vi "Joystick Values To Joystick Data.vi"(0 "Xbox Name":string="My Joystick RefNum", 3 "Left X3D Joystick Name":string="My Joystick RefNum", 5 "Right X3D Joystick Name":string="My Joystick RefNum") -> ()   [LabVIEW 2016]
uses:
  Joystick Global 6740.vi
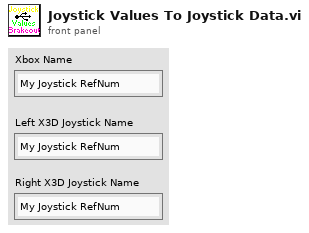
[diagram p1: front panel]
types:
  T1 = cluster{"A":bool, "B":bool, "X":bool, "Y":bool, "LB":bool, "RB":bool, "Back":bool, "Start":bool, "Left Joystick":bool, "Right Joystick":bool}
  T2 = cluster{"Left X":dbl, "Left Y":dbl, "Left Trigger":dbl, "Right Trigger":dbl, "Right X":dbl, "Right Y":dbl}
  T3 = cluster{"1":bool, "2":bool, "3":bool, "4":bool, "5":bool, "6":bool, "7":bool, "8":bool, "9":bool, "10":bool, "11":bool, "12":bool}
  T4 = cluster{"X Axis":dbl, "Y Axis":dbl, "Z Axis":dbl, "Slider":dbl}
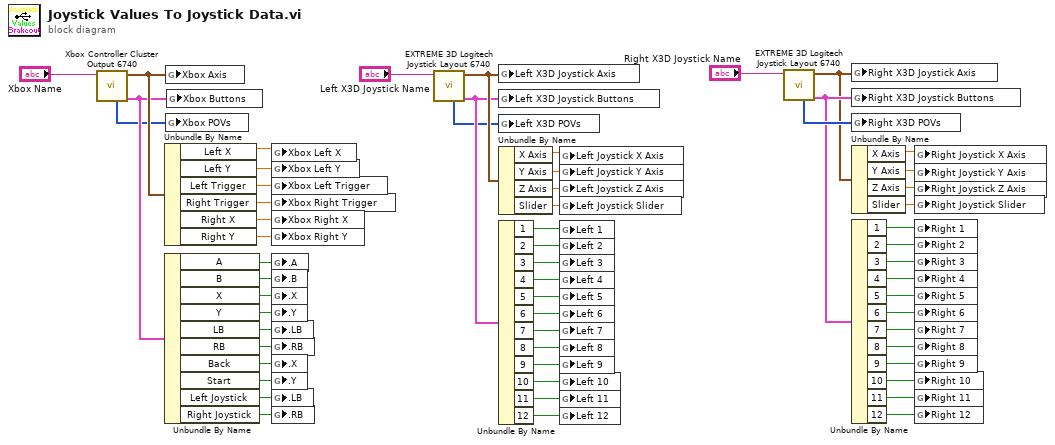
[diagram p0: block diagram]
diagram:
  n1 = call "Xbox Controller Cluster Output 6740.vi"("Joystick Name"="Xbox Name") -> ("Xbox Buttons"=w43:T1, "Xbox Axis"=w44:T2, "POVs"=w21:i16[])  [unwired: 8 in]
  n2 = Unbundle By Name(w44) -> ("Left X"=w60:dbl, "Left Y"=w59:dbl, "Left Trigger"=w58:dbl, "Right Trigger"=w57:dbl, "Right X"=w56:dbl, "Right Y"=w55:dbl)
  n3 = Unbundle By Name(w43) -> ("A"=w54:bool, "B"=w53:bool, "X"=w52:bool, "Y"=w51:bool, "LB"=w50:bool, "RB"=w49:bool, "Back"=w48:bool, "Start"=w47:bool, "Left Joystick"=w46:bool, "Right Joystick"=w45:bool)
  n4 = global write "Joystick Global 6740.vi" "Xbox Axis"(w44) -> ()
  n5 = global write "Joystick Global 6740.vi" "Xbox POVs"(w21) -> ()
  n6 = global write "Joystick Global 6740.vi" "Xbox Buttons"(w43) -> ()
  n7 = global write "Joystick Global 6740.vi" "Xbox Left X"(w60) -> ()
  n8 = global write "Joystick Global 6740.vi" "Xbox Left Y"(w59) -> ()
  n9 = global write "Joystick Global 6740.vi" "Xbox Left Trigger"(w58) -> ()
  n10 = global write "Joystick Global 6740.vi" "Xbox Right Trigger"(w57) -> ()
  n11 = global write "Joystick Global 6740.vi" "Xbox Right X"(w56) -> ()
  n12 = global write "Joystick Global 6740.vi" "Xbox Right Y"(w55) -> ()
  n13 = global write "Joystick Global 6740.vi" ".A"(w54) -> ()
  n14 = global write "Joystick Global 6740.vi" ".B"(w53) -> ()
  n15 = global write "Joystick Global 6740.vi" ".X"(w52) -> ()
  n16 = global write "Joystick Global 6740.vi" ".Y"(w51) -> ()
  n17 = global write "Joystick Global 6740.vi" ".LB"(w50) -> ()
  n18 = global write "Joystick Global 6740.vi" ".RB"(w49) -> ()
  n19 = global write "Joystick Global 6740.vi" ".X"(w48) -> ()
  n20 = global write "Joystick Global 6740.vi" ".Y"(w47) -> ()
  n21 = global write "Joystick Global 6740.vi" ".LB"(w46) -> ()
  n22 = global write "Joystick Global 6740.vi" ".RB"(w45) -> ()
  n23 = call "EXTREME 3D Logitech Joystick Layout 6740.vi"("Joystick Name"="Left X3D Joystick Name") -> ("Logitech Joystick Buttons"=w41:T3, "Logitech Joystick Axis"=w42:T4, "POVs"=w22:i16[])  [unwired: 8 in]
  n24 = global write "Joystick Global 6740.vi" "Left X3D Joystick Axis"(w42) -> ()
  n25 = global write "Joystick Global 6740.vi" "Left X3D Joystick Buttons"(w41) -> ()
  n26 = global write "Joystick Global 6740.vi" "Left X3D POVs"(w22) -> ()
  n27 = Unbundle By Name(w42) -> ("X Axis"=w40:dbl, "Y Axis"=w39:dbl, "Z Axis"=w38:dbl, "Slider"=w37:dbl)
  n28 = Unbundle By Name(w41) -> ("1"=w36:bool, "2"=w35:bool, "3"=w34:bool, "4"=w33:bool, "5"=w32:bool, "6"=w31:bool, "7"=w30:bool, "8"=w29:bool, "9"=w28:bool, "10"=w27:bool, "11"=w26:bool, "12"=w25:bool)
  n29 = global write "Joystick Global 6740.vi" "Left Joystick X Axis"(w40) -> ()
  n30 = global write "Joystick Global 6740.vi" "Left Joystick Y Axis"(w39) -> ()
  n31 = global write "Joystick Global 6740.vi" "Left Joystick Z Axis"(w38) -> ()
  n32 = global write "Joystick Global 6740.vi" "Left Joystick Slider"(w37) -> ()
  n33 = global write "Joystick Global 6740.vi" "Left 1"(w36) -> ()
  n34 = global write "Joystick Global 6740.vi" "Left 2"(w35) -> ()
  n35 = global write "Joystick Global 6740.vi" "Left 3"(w34) -> ()
  n36 = global write "Joystick Global 6740.vi" "Left 4"(w33) -> ()
  n37 = global write "Joystick Global 6740.vi" "Left 5"(w32) -> ()
  n38 = global write "Joystick Global 6740.vi" "Left 6"(w31) -> ()
  n39 = global write "Joystick Global 6740.vi" "Left 7"(w30) -> ()
  n40 = global write "Joystick Global 6740.vi" "Left 8"(w29) -> ()
  n41 = global write "Joystick Global 6740.vi" "Left 9"(w28) -> ()
  n42 = global write "Joystick Global 6740.vi" "Left 10"(w27) -> ()
  n43 = global write "Joystick Global 6740.vi" "Left 11"(w26) -> ()
  n44 = global write "Joystick Global 6740.vi" "Left 12"(w25) -> ()
  n45 = call "EXTREME 3D Logitech Joystick Layout 6740.vi"("Joystick Name"="Right X3D Joystick Name") -> ("Logitech Joystick Buttons"=w2:T3, "Logitech Joystick Axis"=w1:T4, "POVs"=w20:i16[])  [unwired: 8 in]
  n46 = global write "Joystick Global 6740.vi" "Right X3D Joystick Axis"(w1) -> ()
  n47 = global write "Joystick Global 6740.vi" "Right X3D Joystick Buttons"(w2) -> ()
  n48 = global write "Joystick Global 6740.vi" "Right X3D POVs"(w20) -> ()
  n49 = Unbundle By Name(w1) -> ("X Axis"=w3:dbl, "Y Axis"=w4:dbl, "Z Axis"=w5:dbl, "Slider"=w6:dbl)
  n50 = Unbundle By Name(w2) -> ("1"=w7:bool, "2"=w8:bool, "3"=w9:bool, "4"=w10:bool, "5"=w11:bool, "6"=w12:bool, "7"=w13:bool, "8"=w14:bool, "9"=w15:bool, "10"=w16:bool, "11"=w17:bool, "12"=w18:bool)
  n51 = global write "Joystick Global 6740.vi" "Right Joystick X Axis"(w3) -> ()
  n52 = global write "Joystick Global 6740.vi" "Right Joystick Y Axis"(w4) -> ()
  n53 = global write "Joystick Global 6740.vi" "Right Joystick Z Axis"(w5) -> ()
  n54 = global write "Joystick Global 6740.vi" "Right Joystick Slider"(w6) -> ()
  n55 = global write "Joystick Global 6740.vi" "Right 1"(w7) -> ()
  n56 = global write "Joystick Global 6740.vi" "Right 2"(w8) -> ()
  n57 = global write "Joystick Global 6740.vi" "Right 3"(w9) -> ()
  n58 = global write "Joystick Global 6740.vi" "Right 4"(w10) -> ()
  n59 = global write "Joystick Global 6740.vi" "Right 5"(w11) -> ()
  n60 = global write "Joystick Global 6740.vi" "Right 6"(w12) -> ()
  n61 = global write "Joystick Global 6740.vi" "Right 7"(w13) -> ()
  n62 = global write "Joystick Global 6740.vi" "Right 8"(w14) -> ()
  n63 = global write "Joystick Global 6740.vi" "Right 9"(w15) -> ()
  n64 = global write "Joystick Global 6740.vi" "Right 10"(w16) -> ()
  n65 = global write "Joystick Global 6740.vi" "Right 11"(w17) -> ()
  n66 = global write "Joystick Global 6740.vi" "Right 12"(w18) -> ()
